vi "Code da vinci.vi"(8 "error in (no error)":errorcluster, 11 "Cadena entrada":string) -> (0 "error IO":errorcluster, 3 "Codigo":string)   [LabVIEW 2020]
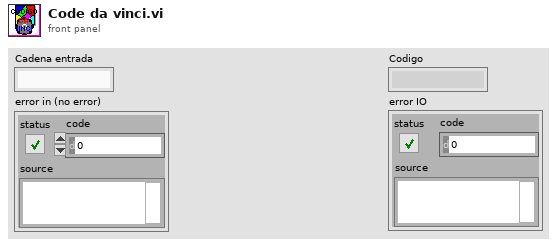
[diagram p1: front panel]
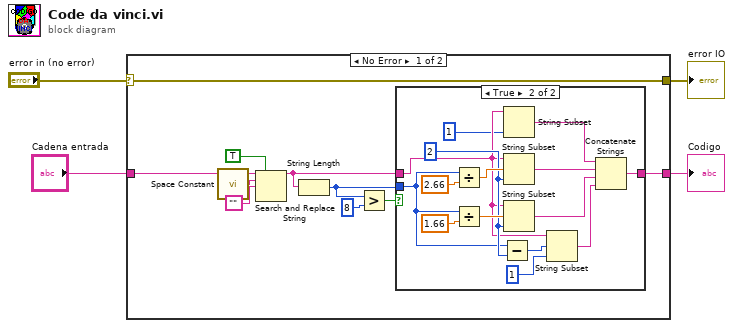
[diagram p0: block diagram]
diagram:
  n1 = case shown="No Error" "error in (no error)" {
    selector: "error in (no error)" -> [w8 w32]
    tunnel: [w14 w31] -> w4
    tunnel: "Cadena entrada" -> [w11 w31]
    tunnel: [w8 w32] -> w1
    frame No Error {
      n2 = call <vilib>:"Space Constant.vi"() -> ("String"=w13:string)
      n3 = Search and Replace String(replace all?=TRUE ("replace all? (F)"), input string=w11, search string=w13, replace string="") -> (result string=w10:string)  [unwired: 4 in, 3 out]
      n4 = String Length(string=w10) -> (length=w7:i32)
      n5 = Greater?(x=w7, y=8) -> (0:w5:bool)
      n6 = case shown="True" w5 {
        tunnel: [w15 w27] -> w14
        tunnel: w10 -> [w15 w21]
        tunnel: w7 -> [_ w18]
        frame False {
        }
        frame True {
          w23 = 2 ("length (rest)")
          n7 = Divide(x=w18, y=2.66) -> (x/y=w24:dbl)
          n8 = Divide(x=w18, y=1.66) -> (x/y=w29:dbl)
          n9 = Subtract(x=w18, y=w23) -> (x-y=w28:i32)
          n10 = String Subset(string=w21, length (rest)=1 ("length (rest)")) -> (substring=w30:string)  [unwired: 1 in]
          n11 = String Subset(string=w21, offset (0)=w24, length (rest)=w23) -> (substring=w20:string)
          n12 = String Subset(string=w21, offset (0)=w29, length (rest)=w23) -> (substring=w19:string)
          n13 = String Subset(string=w21, offset (0)=w28, length (rest)=1 ("length (rest)")) -> (substring=w22:string)
          n14 = Concatenate Strings(w30, w20, w19, w22) -> (w27:string)
        }
      }
    }
    frame Error {
    }
  }
  "Codigo" <- w4
  "error IO" <- w1
